vi "Init.vi"(8 "error in (no error)":errorcluster, 11 "Guardian in":refnum<class "Guardian.lvclass">) -> (0 "error out":errorcluster, 3 "Guardian out":refnum<class "Guardian.lvclass">)   [LabVIEW 2026, in "TALOS.lvlib" / "Guardian.lvlib" / "Guardian.lvclass"]
uses:
  Guardian.lvclass
  Ancestor/Ancestor/Ancestor.lvclass/Ancestor.ctl
  Support VIs/Generate Error.vi
  Support VIs/Circus Root Path.vi
  FGV/Error Memory/Error Memory Core.vi
  FGV/Error Memory/Get Error Description.vi
  Support VIs/Get PC name.vi
  Ancestor/Ancestor/Read ID.vi
  Support VIs/Get Class Name.vi
  <vilib>/Utility/error.llb/Clear Errors.vi
  FGV/Error Memory/Error Crt Lvl checker.vi
  FGV/Error Memory/Error Memory Core.vi/40c8088d-b597-4017-91af-faa98e00292e.vi
  FGV/Error Memory/Error Memory Core.vi/d4a3ab98-063c-4e44-b43d-fbdcfe6c2be2.vi
  <vilib>/AdvancedString/Delimited String to 1D String Array.vi
  <vilib>/AdvancedString/Delimited String to 1D String Array (string).vi
  Support VIs/Global Memory.vi
  <vilib>/Utility/LVClass/Get LV Class Name.vi
  Support VIs/Is in Packed Library.vi
  Support VIs/TALOS Root path.vi
  Support VIs/Read CSV worksheet.vi
  Support VIs/Global Constants.vi
  <vilib>/Utility/error.llb/General Error Handler.vi
  <vilib>/Utility/config.llb/Open Config Data.vi
  <vilib>/Utility/config.llb/Get Section Names.vi
  <vilib>/Utility/config.llb/Get Key Names.vi
  <vilib>/Utility/config.llb/Read Key.vi
  <vilib>/Utility/config.llb/Read Key (String).vi
  <vilib>/Utility/config.llb/Close Config Data.vi
  Ancestor/Ancestor/Ancestor.lvclass
  <vilib>/Comparison/Equal/Equal Functor/Equal Functor.lvclass
  TALOS.lvlib
  FGV/Error Memory/Error Memory.lvlib
  Classes/Error Filter/Error Filter.lvclass
panel:
  out "String":string
  out "Horizontal Progress Bar":u8(slide) scale=0.0..12.0
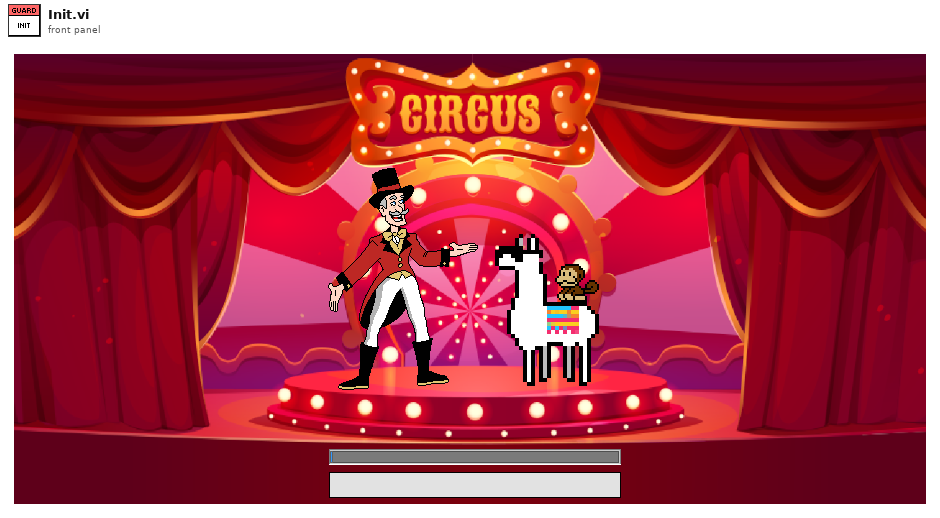
[diagram p1: front panel]
types:
  T1 = enum32{"Invalid", "Standard", "Closed", "Hidden", "Minimized", "Maximized"}
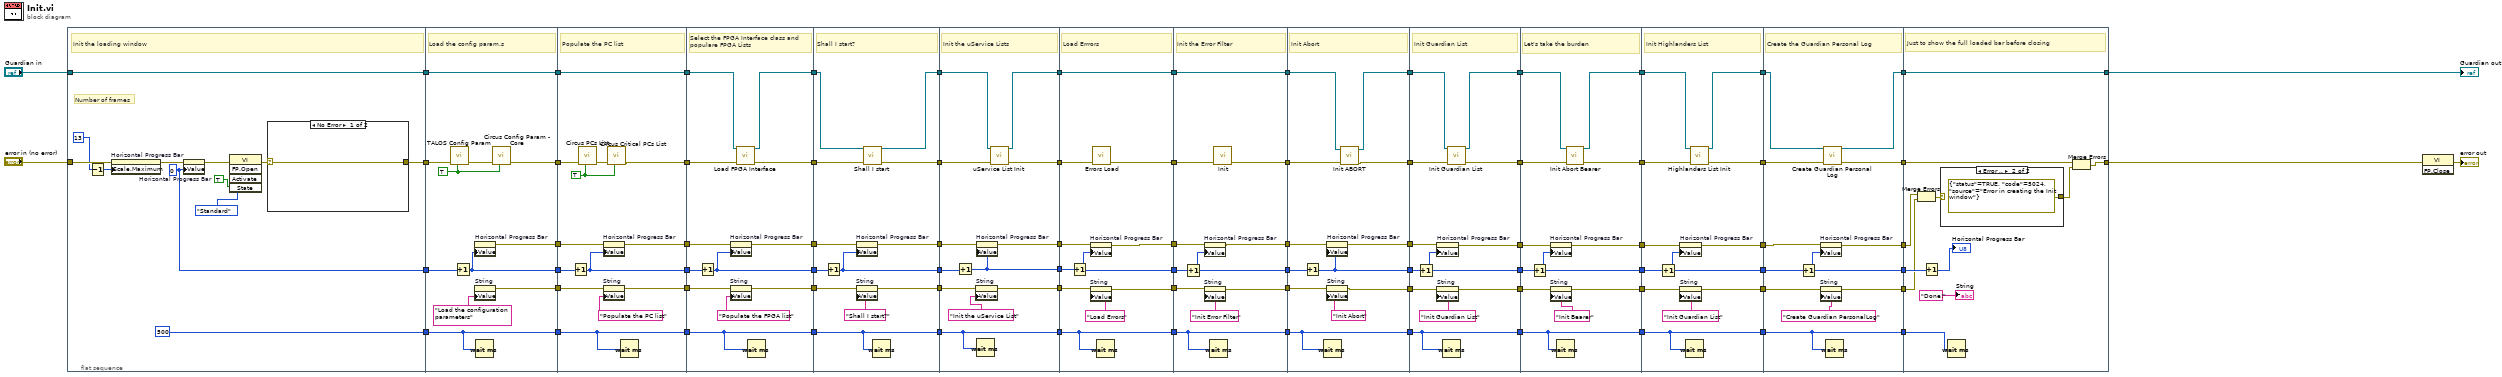
[diagram p0: block diagram]
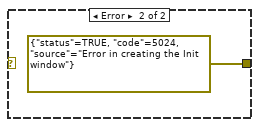
[diagram p2: hidden frame]
diagram:
  n1 = flat-sequence {
    tunnel: "Guardian in" -> [w93]
    tunnel: [w93] -> w4
    tunnel: "error in (no error)" -> [w88]
    tunnel: [w84] -> w3
    tunnel: [w83] -> w2
    tunnel: [u32 500 ("milliseconds to wait")] -> w1
    tunnel: [w101] -> w77
    tunnel: [w106] -> w76
    tunnel: w4 -> [w106]
    tunnel: [w105] -> w75
    tunnel: [w104] -> w74
    tunnel: [w103] -> w73
    tunnel: [w96] -> w66
    tunnel: w3 -> [w97]
    tunnel: w2 -> [w98]
    tunnel: w1 -> [w96]
    tunnel: w77 -> [w112]
    tunnel: [w107] -> w36
    tunnel: w76 -> [w113]
    tunnel: [w113] -> w34
    tunnel: w75 -> [w117]
    tunnel: [w116] -> w32
    tunnel: w74 -> [w119]
    tunnel: [w118] -> w30
    tunnel: w73 -> [w115]
    tunnel: [w111] -> w28
    tunnel: w66 -> [w111]
    tunnel: [w110] -> w26
    tunnel: w36 -> [w123]
    tunnel: [w122] -> w35
    tunnel: w34 -> [w120]
    tunnel: [w121] -> w33
    tunnel: w32 -> [w128]
    tunnel: [w127] -> w31
    tunnel: w30 -> [w130]
    tunnel: [w129] -> w29
    tunnel: w28 -> [w124]
    tunnel: [w124] -> w27
    tunnel: w26 -> [w126]
    tunnel: [w125] -> w25
    tunnel: w35 -> [w134]
    tunnel: [w135] -> w53
    tunnel: w33 -> [w132]
    tunnel: [w133] -> w52
    tunnel: w31 -> [w139]
    tunnel: w29 -> [w137]
    tunnel: [w136] -> w51
    tunnel: w27 -> [w140]
    tunnel: [w140] -> w50
    tunnel: w25 -> [w142]
    tunnel: [w141] -> w49
    tunnel: [w138] -> w48
    tunnel: w53 -> [w155]
    tunnel: w52 -> [w145]
    tunnel: [w146] -> w72
    tunnel: w51 -> [w154]
    tunnel: [w153] -> w71
    tunnel: [w149] -> w70
    tunnel: [w148] -> w69
    tunnel: [w151] -> w68
    tunnel: [w147] -> w67
    tunnel: w50 -> [w147]
    tunnel: w49 -> [w144]
    tunnel: w48 -> [w152]
    tunnel: w72 -> [w166]
    tunnel: [w166] -> w65
    tunnel: w71 -> [w160]
    tunnel: w70 -> [w164]
    tunnel: [w163] -> w63
    tunnel: w69 -> [w158]
    tunnel: [w157] -> w61
    tunnel: w68 -> [w162]
    tunnel: [w161] -> w59
    tunnel: [w159] -> w57
    tunnel: [w156] -> w55
    tunnel: w67 -> [w156]
    tunnel: w65 -> [w177]
    tunnel: [w177] -> w64
    tunnel: w63 -> [w174]
    tunnel: [w175] -> w62
    tunnel: w61 -> [w167]
    tunnel: [w168] -> w60
    tunnel: w59 -> [w172]
    tunnel: [w171] -> w58
    tunnel: w57 -> [w169]
    tunnel: [w170] -> w56
    tunnel: w55 -> [w173]
    tunnel: [w173] -> w54
    tunnel: w64 -> [w184]
    tunnel: w62 -> [w187]
    tunnel: w60 -> [w185]
    tunnel: w58 -> [w189]
    tunnel: w56 -> [w188]
    tunnel: w54 -> [w178]
    tunnel: [w183] -> w10
    tunnel: [w182] -> w9
    tunnel: [w181] -> w8
    tunnel: [w180] -> w7
    tunnel: [w179] -> w6
    tunnel: [w178] -> w5
    tunnel: w10 -> [w196]
    tunnel: [w197] -> w24
    tunnel: [w195] -> w22
    tunnel: [w200] -> w20
    tunnel: [w199] -> w19
    tunnel: [w198] -> w18
    tunnel: [w190] -> w17
    tunnel: w9 -> [w194]
    tunnel: w8 -> [w193]
    tunnel: w7 -> [w192]
    tunnel: w6 -> [w191]
    tunnel: w5 -> [w190]
    tunnel: w24 -> [w210]
    tunnel: [w211] -> w23
    tunnel: w22 -> [w212]
    tunnel: [w213] -> w21
    tunnel: w20 -> [w208]
    tunnel: w19 -> [w204]
    tunnel: w18 -> [w206]
    tunnel: w17 -> [w202]
    tunnel: [w207] -> w16
    tunnel: [w205] -> w15
    tunnel: [w203] -> w14
    tunnel: [w202] -> w11
    tunnel: w23 -> [w220]
    tunnel: [w221] -> w46
    tunnel: w21 -> [w218]
    tunnel: [w219] -> w44
    tunnel: [w223] -> w42
    tunnel: [w222] -> w40
    tunnel: [w224] -> w38
    tunnel: w16 -> [w217]
    tunnel: w15 -> [w216]
    tunnel: w14 -> [w215]
    tunnel: [w214] -> w12
    tunnel: w11 -> [w214]
    tunnel: w46 -> [w229]
    tunnel: [w230] -> w45
    tunnel: w44 -> [w228]
    tunnel: [w227] -> w43
    tunnel: w42 -> [w235]
    tunnel: [w236] -> w41
    tunnel: w40 -> [w233]
    tunnel: [w234] -> w39
    tunnel: w38 -> [w231]
    tunnel: [w232] -> w37
    tunnel: [w226] -> w13
    tunnel: w12 -> [w226]
    tunnel: [w246] -> w79
    tunnel: w45 -> [w248]
    tunnel: [w248] -> w81
    tunnel: w43 -> [w244]
    tunnel: w41 -> [w242]
    tunnel: w39 -> [w243]
    tunnel: w37 -> [w241]
    tunnel: w13 -> [w238]
    frame #0 {
      w83 = u8 0 ("Slide")
      # "Number of frames"
      # "Init the loading window"
      n2 = Decrement(x=u8 13 ("Slide")) -> (x-1=w86:u8)
      n3 = property on="Horizontal Progress Bar" class="Slide (strict)"(error in=w88, "Scale.Maximum"=w86) -> (error out=w89:errorcluster)  [unwired: 1 in, 1 out]
      n4 = property on="Horizontal Progress Bar" class="Slide (strict)"(error in=w89, "Value"=w83) -> (error out=w92:errorcluster)  [unwired: 1 in, 1 out]
      n5 = invoke class="VI" method="FP.Open"(error in=w92, "Activate"=TRUE ("Activate?"), "State"=T1."Standard") -> (error out=w85:errorcluster)  [unwired: 2 in, 4 out]
      n6 = case shown="No Error" w85 {
        selector: w85 -> [w94 _]
        tunnel: [w94 errorcluster {"status"=TRUE, "code"=5024, "source"="Error in creating the Init window"} ("error IO")] -> w84
        frame No Error {
        }
        frame Error {
        }
      }
    }
    frame #1 {
      w99 = TRUE ("Load")
      # "Load the config param.s"
      n7 = call "TALOS Config Param.vi"("Load"=w99, "error in (no error)"=w97) -> ("error out"=w100:errorcluster)  [unwired: 8 in, 1 out]
      n8 = Increment(x=w98) -> (x+1=w105:u8)
      n9 = property on="Horizontal Progress Bar" class="Slide (strict)"("Value"=w105) -> (error out=w104:errorcluster)  [unwired: 2 in, 1 out]
      n10 = property on="String" class="Str"("Value"="Load the configuration parameters" ("String")) -> (error out=w103:errorcluster)  [unwired: 2 in, 1 out]
      n11 = Wait (ms)(milliseconds to wait=w96) -> ()  [unwired: 1 out]
      n12 = call "Circus Config Param - Core.vi"("Load"=w99, "error in (no error)"=w100) -> ("error out"=w101:errorcluster)  [unwired: 8 in, 1 out]
    }
    frame #2 {
      w108 = TRUE ("Init")
      # "Populate the PC list"
      n13 = Increment(x=w117) -> (x+1=w116:u8)
      n14 = call "Circus PCs List.vi"("Init"=w108, "error in (no error)"=w112) -> ("error out"=w109:errorcluster)  [unwired: 8 in, 1 out]
      n15 = property on="Horizontal Progress Bar" class="Slide (strict)"(error in=w119, "Value"=w116) -> (error out=w118:errorcluster)  [unwired: 1 in, 1 out]
      n16 = property on="String" class="Str"(error in=w115, "Value"="Populate the PC list" ("String")) -> (error out=w110:errorcluster)  [unwired: 1 in, 1 out]
      n17 = call "Circus Critical PCs List.vi"("Init"=w108, "error in (no error)"=w109) -> ("error out"=w107:errorcluster)  [unwired: 8 in, 1 out]
      n18 = Wait (ms)(milliseconds to wait=w111) -> ()  [unwired: 1 out]
    }
    frame #3 {
      # "Select the FPGA Interface class and populare FPGA Lists"
      n19 = Increment(x=w128) -> (x+1=w127:u8)
      n20 = property on="Horizontal Progress Bar" class="Slide (strict)"(error in=w130, "Value"=w127) -> (error out=w129:errorcluster)  [unwired: 1 in, 1 out]
      n21 = property on="String" class="Str"(error in=w126, "Value"="Populate the FPGA list" ("String")) -> (error out=w125:errorcluster)  [unwired: 1 in, 1 out]
      n22 = call "Load FPGA Interface.vi"("error in (no error)"=w123, "Guardian in"=w120) -> ("error out"=w122:errorcluster, "Guardian out"=w121:refnum<class "Guardian.lvclass">)  [unwired: 8 in]
      n23 = Wait (ms)(milliseconds to wait=w124) -> ()  [unwired: 1 out]
    }
    frame #4 {
      # "Shall I start?"
      n24 = Increment(x=w139) -> (x+1=w138:u8)
      n25 = property on="Horizontal Progress Bar" class="Slide (strict)"(error in=w137, "Value"=w138) -> (error out=w136:errorcluster)  [unwired: 1 in, 1 out]
      n26 = property on="String" class="Str"(error in=w142, "Value"="Shall I start?" ("String")) -> (error out=w141:errorcluster)  [unwired: 1 in, 1 out]
      n27 = call "Shall I start.vi"("error in (no error)"=w134, "Guardian in"=w132) -> ("error out"=w135:errorcluster, "Guardian out"=w133:refnum<class "Guardian.lvclass">)  [unwired: 8 in]
      n28 = Wait (ms)(milliseconds to wait=w140) -> ()  [unwired: 1 out]
    }
    frame #5 {
      # "Init the uService Lists"
      n29 = Increment(x=w152) -> (x+1=w151:u8)
      n30 = property on="String" class="Str"(error in=w144, "Value"="Init the uService List" ("String")) -> (error out=w149:errorcluster)  [unwired: 1 in, 1 out]
      n31 = property on="Horizontal Progress Bar" class="Slide (strict)"(error in=w154, "Value"=w151) -> (error out=w153:errorcluster)  [unwired: 1 in, 1 out]
      n32 = Wait (ms)(milliseconds to wait=w147) -> ()  [unwired: 1 out]
      n33 = call "uService List Init.vi"("error in (no error)"=w155, "Guardian in"=w145) -> ("error out"=w148:errorcluster, "Guardian out"=w146:refnum<class "Guardian.lvclass">)  [unwired: 8 in]
    }
    frame #6 {
      # "Load Errrors"
      n34 = Increment(x=w162) -> (x+1=w161:u8)
      n35 = property on="Horizontal Progress Bar" class="Slide (strict)"(error in=w160, "Value"=w161) -> (error out=w159:errorcluster)  [unwired: 1 in, 1 out]
      n36 = property on="String" class="Str"(error in=w164, "Value"="Load Errors" ("String")) -> (error out=w163:errorcluster)  [unwired: 1 in, 1 out]
      n37 = call "Errors Load.vi"("error in (no error)"=w158) -> ("error out"=w157:errorcluster)  [unwired: 10 in]
      n38 = Wait (ms)(milliseconds to wait=w156) -> ()  [unwired: 1 out]
    }
    frame #7 {
      # "Init the Error Filter"
      n39 = Increment(x=w172) -> (x+1=w171:u8)
      n40 = property on="Horizontal Progress Bar" class="Slide (strict)"(error in=w169, "Value"=w171) -> (error out=w170:errorcluster)  [unwired: 1 in, 1 out]
      n41 = property on="String" class="Str"(error in=w174, "Value"="Init Error Filter" ("String")) -> (error out=w175:errorcluster)  [unwired: 1 in, 1 out]
      n42 = Wait (ms)(milliseconds to wait=w173) -> ()  [unwired: 1 out]
      n43 = call "Init.vi"("error in (no error)"=w167) -> ("error out"=w168:errorcluster)  [unwired: 10 in]
    }
    frame #8 {
      # "Init Abort"
      n44 = Increment(x=w189) -> (x+1=w180:u8)
      n45 = Wait (ms)(milliseconds to wait=w178) -> ()  [unwired: 1 out]
      n46 = property on="Horizontal Progress Bar" class="Slide (strict)"(error in=w188, "Value"=w180) -> (error out=w181:errorcluster)  [unwired: 1 in, 1 out]
      n47 = property on="String" class="Str"(error in=w187, "Value"="Init Abort" ("String")) -> (error out=w179:errorcluster)  [unwired: 1 in, 1 out]
      n48 = call "Init ABORT.vi"("error in (no error)"=w185, "Guardian in"=w184) -> ("error out"=w182:errorcluster, "Guardian out"=w183:refnum<class "Guardian.lvclass">)  [unwired: 8 in]
    }
    frame #9 {
      # "Init Guardian List"
      n49 = Increment(x=w192) -> (x+1=w199:u8)
      n50 = property on="Horizontal Progress Bar" class="Slide (strict)"(error in=w193, "Value"=w199) -> (error out=w200:errorcluster)  [unwired: 1 in, 1 out]
      n51 = property on="String" class="Str"(error in=w191, "Value"="Init Guardian List" ("String")) -> (error out=w198:errorcluster)  [unwired: 1 in, 1 out]
      n52 = Wait (ms)(milliseconds to wait=w190) -> ()  [unwired: 1 out]
      n53 = call "Init Guardian List.vi"("error in (no error)"=w194, "Guardian in"=w196) -> ("error out"=w195:errorcluster, "Guardian out"=w197:refnum<class "Guardian.lvclass">)  [unwired: 8 in]
    }
    frame #10 {
      # "Let's take the burden"
      n54 = Increment(x=w204) -> (x+1=w203:u8)
      n55 = property on="Horizontal Progress Bar" class="Slide (strict)"(error in=w208, "Value"=w203) -> (error out=w207:errorcluster)  [unwired: 1 in, 1 out]
      n56 = property on="String" class="Str"(error in=w206, "Value"="Init Bearer" ("String")) -> (error out=w205:errorcluster)  [unwired: 1 in, 1 out]
      n57 = Wait (ms)(milliseconds to wait=w202) -> ()  [unwired: 1 out]
      n58 = call "Init Abort Bearer.vi"("error in (no error)"=w212, "Guardian in"=w210) -> ("error out"=w213:errorcluster, "Guardian out"=w211:refnum<class "Guardian.lvclass">)  [unwired: 8 in]
    }
    frame #11 {
      # "Init Highlanders List"
      n59 = Increment(x=w215) -> (x+1=w222:u8)
      n60 = property on="Horizontal Progress Bar" class="Slide (strict)"(error in=w217, "Value"=w222) -> (error out=w223:errorcluster)  [unwired: 1 in, 1 out]
      n61 = property on="String" class="Str"(error in=w216, "Value"="Init Guardian List" ("String")) -> (error out=w224:errorcluster)  [unwired: 1 in, 1 out]
      n62 = Wait (ms)(milliseconds to wait=w214) -> ()  [unwired: 1 out]
      n63 = call "Highlanders List Init.vi"("error in (no error)"=w218, "Guardian in"=w220) -> ("error out"=w219:errorcluster, "Guardian out"=w221:refnum<class "Guardian.lvclass">)  [unwired: 8 in]
    }
    frame #12 {
      # "Create the Guardian Personal Log"
      n64 = Increment(x=w233) -> (x+1=w234:u8)
      n65 = property on="Horizontal Progress Bar" class="Slide (strict)"(error in=w235, "Value"=w234) -> (error out=w236:errorcluster)  [unwired: 1 in, 1 out]
      n66 = property on="String" class="Str"(error in=w231, "Value"="Create Guardian PersonalLog" ("String")) -> (error out=w232:errorcluster)  [unwired: 1 in, 1 out]
      n67 = call "Create Guardian Personal Log.vi"("error in (no error)"=w228, "Guardian in"=w229) -> ("error out"=w227:errorcluster, "Guardian out"=w230:refnum<class "Guardian.lvclass">)  [unwired: 8 in]
      n68 = Wait (ms)(milliseconds to wait=w226) -> ()  [unwired: 1 out]
    }
    frame #13 {
      # "Just to show the full loaded bar before closing"
      n69 = Merge Errors(w242, w241) -> (w239:errorcluster)
      n70 = Increment(x=w243) -> (x+1=→"Horizontal Progress Bar":u8)
      n71 = case shown="Error .." w239 {
        selector: w239 -> [w249 _]
        tunnel: [w249 errorcluster {"status"=TRUE, "code"=5024, "source"="Error in creating the Init window"} ("error IO")] -> w240
        frame No Error {
        }
        frame Error {
        }
      }
      n72 = Wait (ms)(milliseconds to wait=w238) -> ()  [unwired: 1 out]
      n73 = Merge Errors(w244, w240) -> (w246:errorcluster)
      "String" <- "Done!" ("String")
    }
  }
  n74 = invoke class="VI" method="FP.Close"(error in=w79) -> (error out=→"error out":errorcluster)  [unwired: 2 in, 2 out]
  "Guardian out" <- w81
